vi "Get Tunnel Diagrams_Flat Sequence.vi"(7 "Tunnel Type":enum16{"Tunnel", "FlatSeqInner", "FlatSeqOuter"}(ring), 8 "error in":errorcluster, 10 "FlatSeqOutTun Refnum":refnum<vi>, 11 "FlatSeqInTun Refnum":refnum<vi>) -> (0 "error out":errorcluster, 1 "Inner Diagram found?":bool, 2 "Inner/Right Diagram":refnum<vi>, 3 "Outer/Left Diagram":refnum<vi>, 4 "Inner/Right Terminal":refnum<vi>, 5 "Outer/Left Terminal":refnum<vi>)   [LabVIEW 2023]
doc: "Returns the outer diagram and inner diagram references for a tunnel. the inner will be the currently displayed frame on a multi-frame structure, suce as an event or case structure.\n\nOuter diagram is the diagram reference for outside the structure. It is the Left diagram for an inner terminal tunnel of a flat sequence structure.\n\nInner diagram is the reference to the diagram inside the structure. It is the right-side diagram for an inner terminal tunnel of a flat sequence structure."
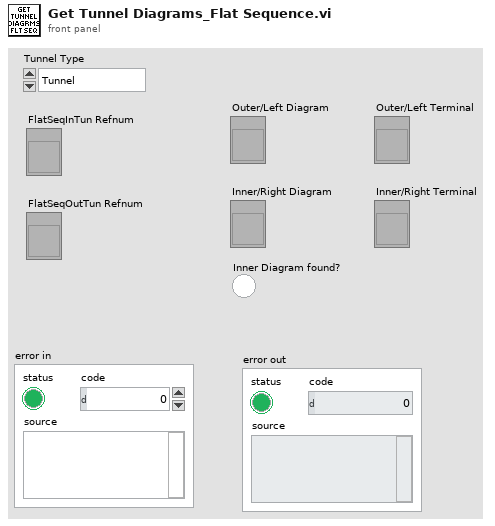
[diagram p1: front panel]
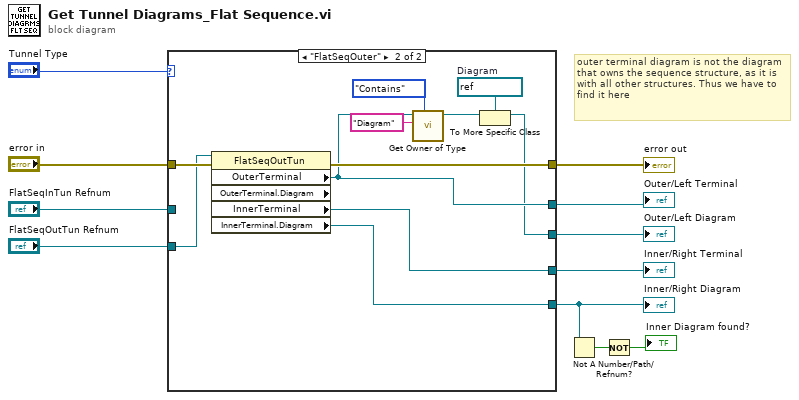
[diagram p0: block diagram]
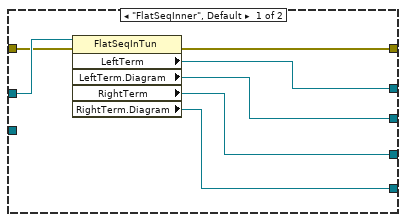
[diagram p2: hidden frame]
diagram:
  # "outer terminal diagram is not the diagram that owns the sequence structure, as it is with all other structures. Thus we have to find it here"
  n1 = case shown="\"FlatSeqOuter\"" "Tunnel Type" {
    tunnel: [w17 w20] -> w11
    tunnel: [w12 w26] -> w2
    tunnel: "error in" -> [w15 w29]
    tunnel: "FlatSeqInTun Refnum" -> [w18 _]
    tunnel: "FlatSeqOutTun Refnum" -> [_ w28]
    tunnel: [w16 w25] -> w6
    tunnel: [w14 w22] -> w5
    tunnel: [w13 w27] -> w4
    frame "FlatSeqInner", Default {
      n2 = property class="FlatSeqInTun"(reference=w18, error in=w15) -> (error out=w16:errorcluster, "LeftTerm"=w14:refnum<vi>, "LeftTerm.Diagram"=w17:refnum<vi>, "RightTerm"=w13:refnum<vi>, "RightTerm.Diagram"=w12:refnum<vi>)  [unwired: 1 out]
    }
    frame "FlatSeqOuter" {
      w19 = refnum<vi> refnum  # Diagram
      n3 = property class="FlatSeqOutTun" props=["OuterTerminal", "OuterTerminal", "Diagram", "InnerTerminal", "InnerTerminal", "Diagram"](reference=w28, error in=w29) -> (error out=w25:errorcluster, "OuterTerminal"=w22:refnum<vi>, "InnerTerminal"=w27:refnum<vi>, "InnerTerminal.Diagram"=w26:refnum<vi>)  [unwired: 2 out]
      n4 = call "Get Owner of Type.vi"("Match Type"=enum16{"Exact Match", "Contains"}."Contains", "Owner Class Name desired"="Diagram", "reference"=w22) -> ("Owner of Type"=w21:refnum<vi>)  [unwired: 4 in, 4 out]
      n5 = To More Specific Class(target class=w19, reference=w21) -> (specific class reference=w20:refnum<vi>)  [unwired: 1 in, 1 out]
    }
  }
  "Inner/Right Diagram" <- w2
  "Outer/Left Diagram" <- w11
  "error out" <- w6
  "Outer/Left Terminal" <- w5
  "Inner/Right Terminal" <- w4
  n6 = Not A Number/Path/Refnum?(number/path/refnum=w2) -> (NaN/Path/Refnum?=w3:bool)
  n7 = Not(x=w3) -> (.not. x?=→"Inner Diagram found?":bool)
